vi "Configure Frequency.vi"(7 "Mode":enum16{"Center Span", "Start Stop"}(ring), 8 "error in (no error)":errorcluster, 9 "Span/Stop Frequency":dbl, 10 "Center/Start Frequency":dbl, 11 "VNA-Keysight PNA in":refnum<class "VNA-Keysight PNA.lvclass">) -> (0 "error out":errorcluster, 3 "VNA-Keysight PNA out":refnum<class "VNA-Keysight PNA.lvclass">)   [LabVIEW 2020, in "VNA-Keysight PNA.lvclass"]
doc: "Configures the frequency range for the sweep.\nThe default mode is Center Span."
uses:
  VNA-Keysight PNA.lvclass
  C:/Sandbox/Git_Sandbox/WiSpry Test Framework source code (LV20)/WiSpry Test Framework/Instruments/Vector Network Analyzer/Vector Network Analyzer.lvclass
  C:/Sandbox/Git_Sandbox/WiSpry Test Framework source code (LV20)/WiSpry Test Framework/Instruments/Instrument.lvclass
  Instrument.lvclass/Instrument.ctl
  Vector Network Analyzer.lvclass/Vector Network Analyzer.ctl
  Instrument.lvclass
  <instrlib>/Keysight PNA Series/Keysight PNA Series.lvlib
  Vector Network Analyzer.lvclass
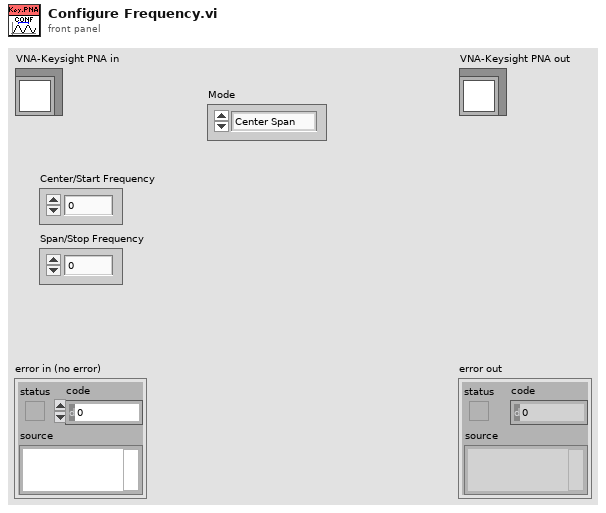
[diagram p1: front panel]
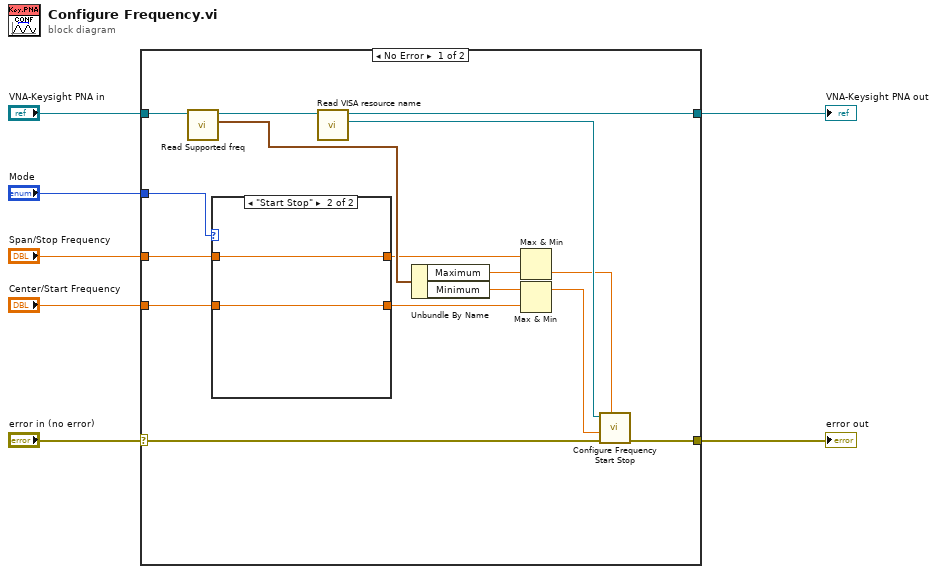
[diagram p0: block diagram]
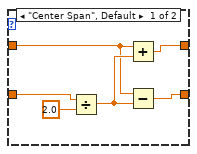
[diagram p2: hidden frame]
diagram:
  n1 = case shown="No Error" "error in (no error)" {
    selector: "error in (no error)" -> [w22 w32]
    tunnel: [w23 w33] -> w5
    tunnel: "VNA-Keysight PNA in" -> [w16 w33]
    tunnel: [w21 w32] -> w6
    tunnel: "Span/Stop Frequency" -> [w18 _]
    tunnel: "Center/Start Frequency" -> [w17 _]
    tunnel: "Mode" -> [w19 _]
    frame No Error {
      n2 = call "Read Supported freq.vi"("Vector Network Analyzer in"=w16) -> ("Supported freq"=w14:cluster{"Minimum":dbl, "Maximum":dbl}, "Vector Network Analyzer out"=w15:refnum<class "VNA-Keysight PNA.lvclass">)  [unwired: 9 in]
      n3 = case shown="\"Start Stop\"" w19 {
        tunnel: [w29 w31] -> w11
        tunnel: w18 -> [w24 w31]
        tunnel: [w28 w30] -> w10
        tunnel: w17 -> [w27 w30]
        frame "Center Span", Default {
          n4 = Divide(x=w27, y=2.0) -> (x/y=w25:dbl)
          n5 = Add(x=w24, y=w25) -> (x+y=w29:dbl)
          n6 = Subtract(x=w24, y=w25) -> (x-y=w28:dbl)
        }
        frame "Start Stop" {
        }
      }
      n7 = call "Read VISA resource name.vi"("Instrument in"=w15) -> ("VISA resource name"=w20:refnum<visa-resource-name>, "Instrument out"=w23:refnum<class "VNA-Keysight PNA.lvclass">)  [unwired: 9 in]
      n8 = Unbundle By Name(w14) -> ("Maximum"=w12:dbl, "Minimum"=w13:dbl)
      n9 = Max & Min(x=w11, y=w12) -> (min(x,y)=w8:dbl)  [unwired: 1 out]
      n10 = Max & Min(x=w13, y=w10) -> (max(x,y)=w9:dbl)  [unwired: 1 out]
      n11 = call <instrlib>:"Configure Frequency Start Stop.vi"("Stop Frequency (2E+6 Hz)"=w8, "error in (no error)"=w22, "Start Frequency (1E+6 Hz)"=w9, "VISA resource name"=w20) -> ("error out"=w21:errorcluster)  [unwired: 6 in, 1 out]
    }
    frame Error {
    }
  }
  "error out" <- w6
  "VNA-Keysight PNA out" <- w5
